vi "Verify TestStand Availability.vi"(11 "error in":errorcluster) -> (4 "test stand installed?":bool, 15 "error out":errorcluster)   [LabVIEW 2021, in "Create Sequence.lvlib"]
uses:
  Create Sequence.lvlib
  <vilib>/nisyscfg/Get Installed Components.vi
  <vilib>/nisyscfg/Close (System).vi
  <vilib>/nisyscfg/nisyscfg.lvlib
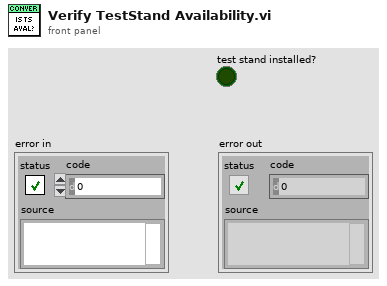
[diagram p1: front panel]
types:
  T1 = typedef "nisyscfg.lvlib/Software 1.2.ctl" = cluster{"title":string, "description":string, "ID":string, "version":string, "component type":T2}
  T2 = typedef "nisyscfg.lvlib/Component Type.ctl" = u32
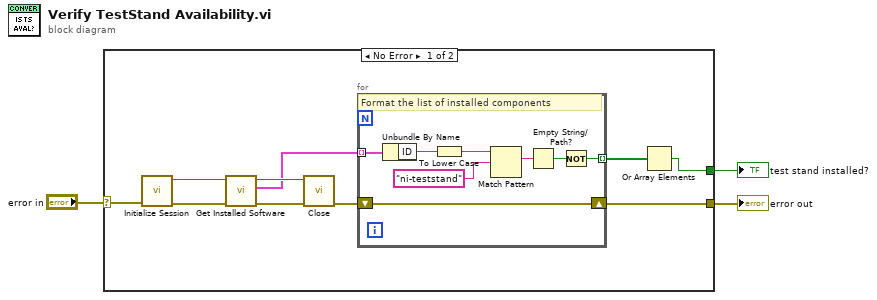
[diagram p0: block diagram]
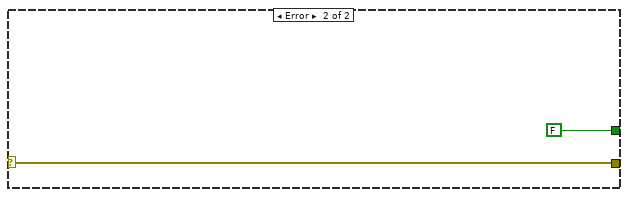
[diagram p2: hidden frame]
diagram:
  n1 = case shown="No Error" "error in" {
    selector: "error in" -> [w7 w23]
    tunnel: [w4 FALSE] -> w3
    tunnel: [w6 w23] -> w1
    frame No Error {
      n2 = call <vilib>:"Initialize Session.vi"("error in (no error)"=w7) -> ("error out"=w13:errorcluster, "Session out"=w12:refnum<k21>)  [unwired: 9 in]
      n3 = call-poly <vilib>:"Get Installed Software.vi"("error in (no error)"=w13, "Session in"=w12) -> ("error out"=w11:errorcluster, "Software Components"=w9:T1[], "Session out"=w10:refnum<k21>)  [unwired: 7 in]
      n4 = call-poly <vilib>:"Close.vi"("error in (no error)"=w11, "Session in"=w10) -> ("error out"=w8:errorcluster)  [unwired: 9 in]
      n5 = for {
        tunnel: w9 -> [w21] mode=indexing
        shift-right: [w17] -> w6
        shift-left: w8 -> [w17]
        tunnel: [w14] -> w5 mode=indexing
        # "Format the list of installed components"
        n6 = Unbundle By Name(w21) -> ("ID"=w20:string)
        n7 = To Lower Case(string=w20) -> (all lower case string=w19:string)
        n8 = Match Pattern(string=w19, regular expression="ni-teststand") -> (match substring=w16:string)  [unwired: 1 in, 3 out]
        n9 = Empty String/Path?(string/path=w16) -> (empty?=w15:bool)
        n10 = Not(x=w15) -> (.not. x?=w14:bool)
      }
      n11 = Or Array Elements(Boolean array=w5) -> (logical OR=w4:bool)
    }
    frame Error {
    }
  }
  "test stand installed?" <- w3
  "error out" <- w1
